vi "zgj地图的构建0911-150原.vi"() -> ()   [LabVIEW 2018]
uses:
  <vilib>/Utility/file.llb/Read Delimited Spreadsheet (string).vi
  <vilib>/vision/NI_Vision_Development_Module.lvlib
panel:
  out "方向":sgl
  out "轨迹跟踪点数":i32
  out "y":dbl
  out "x":dbl
  out "b":dbl[](array[numeric])
  in  "pp":dbl
  out "与目标点的距离":sgl
  in  "guiji":path=path "G:/ICRA-2024-Yuezhen Liu/Labview程序-ICRA2024-YuezhenLiu/small_myRIO_Helmholtz - 1111ke777/zgj轨迹delta为150.txt" caption="call7-8"
  out "i":i32
  out "Image 7":T1(plugin-control)
  in  "Stop (F)":bool
  out "数值 2":dbl
  out "数值":dbl
  out "数组":sgl[](array[numeric])
  out "Objects":T2(array[cluster]) {"Aspect Ratio" format="%.2f"; "Orientation" format="%.2f"; "Area" format="%.2f"; "Object Center"."Y" format="%.2f"; "Object Center"."X" format="%.2f"}
  in  "Settings":T3={"Objects"=0, "Threshold"=128, "Reject Border"=FALSE, "Fill Holes"=FALSE, "Min Object Size"=TRUE, "Min Size"=5000, "Max Object Size"=FALSE, "Max Size"=100, "Show Search Area"=FALSE, "Show Center"=TRUE, "Show Bounding Box"=TRUE} {"Objects" items=["Bright Objects", "Dark Objects"]; "Threshold" min=1 max=999999999 step=1; "Max Size" min=1 max=999999999 step=1; "Min Size" min=1 max=999999999 step=1}
  out "Image 2":T1(plugin-control)
  in  "Range":cluster{"Lower value":sgl, "Upper value":sgl}={"Lower value"=0.0, "Upper value"=128.0} {"Upper value" format="%.2f"; "Lower value" format="%.2f"}
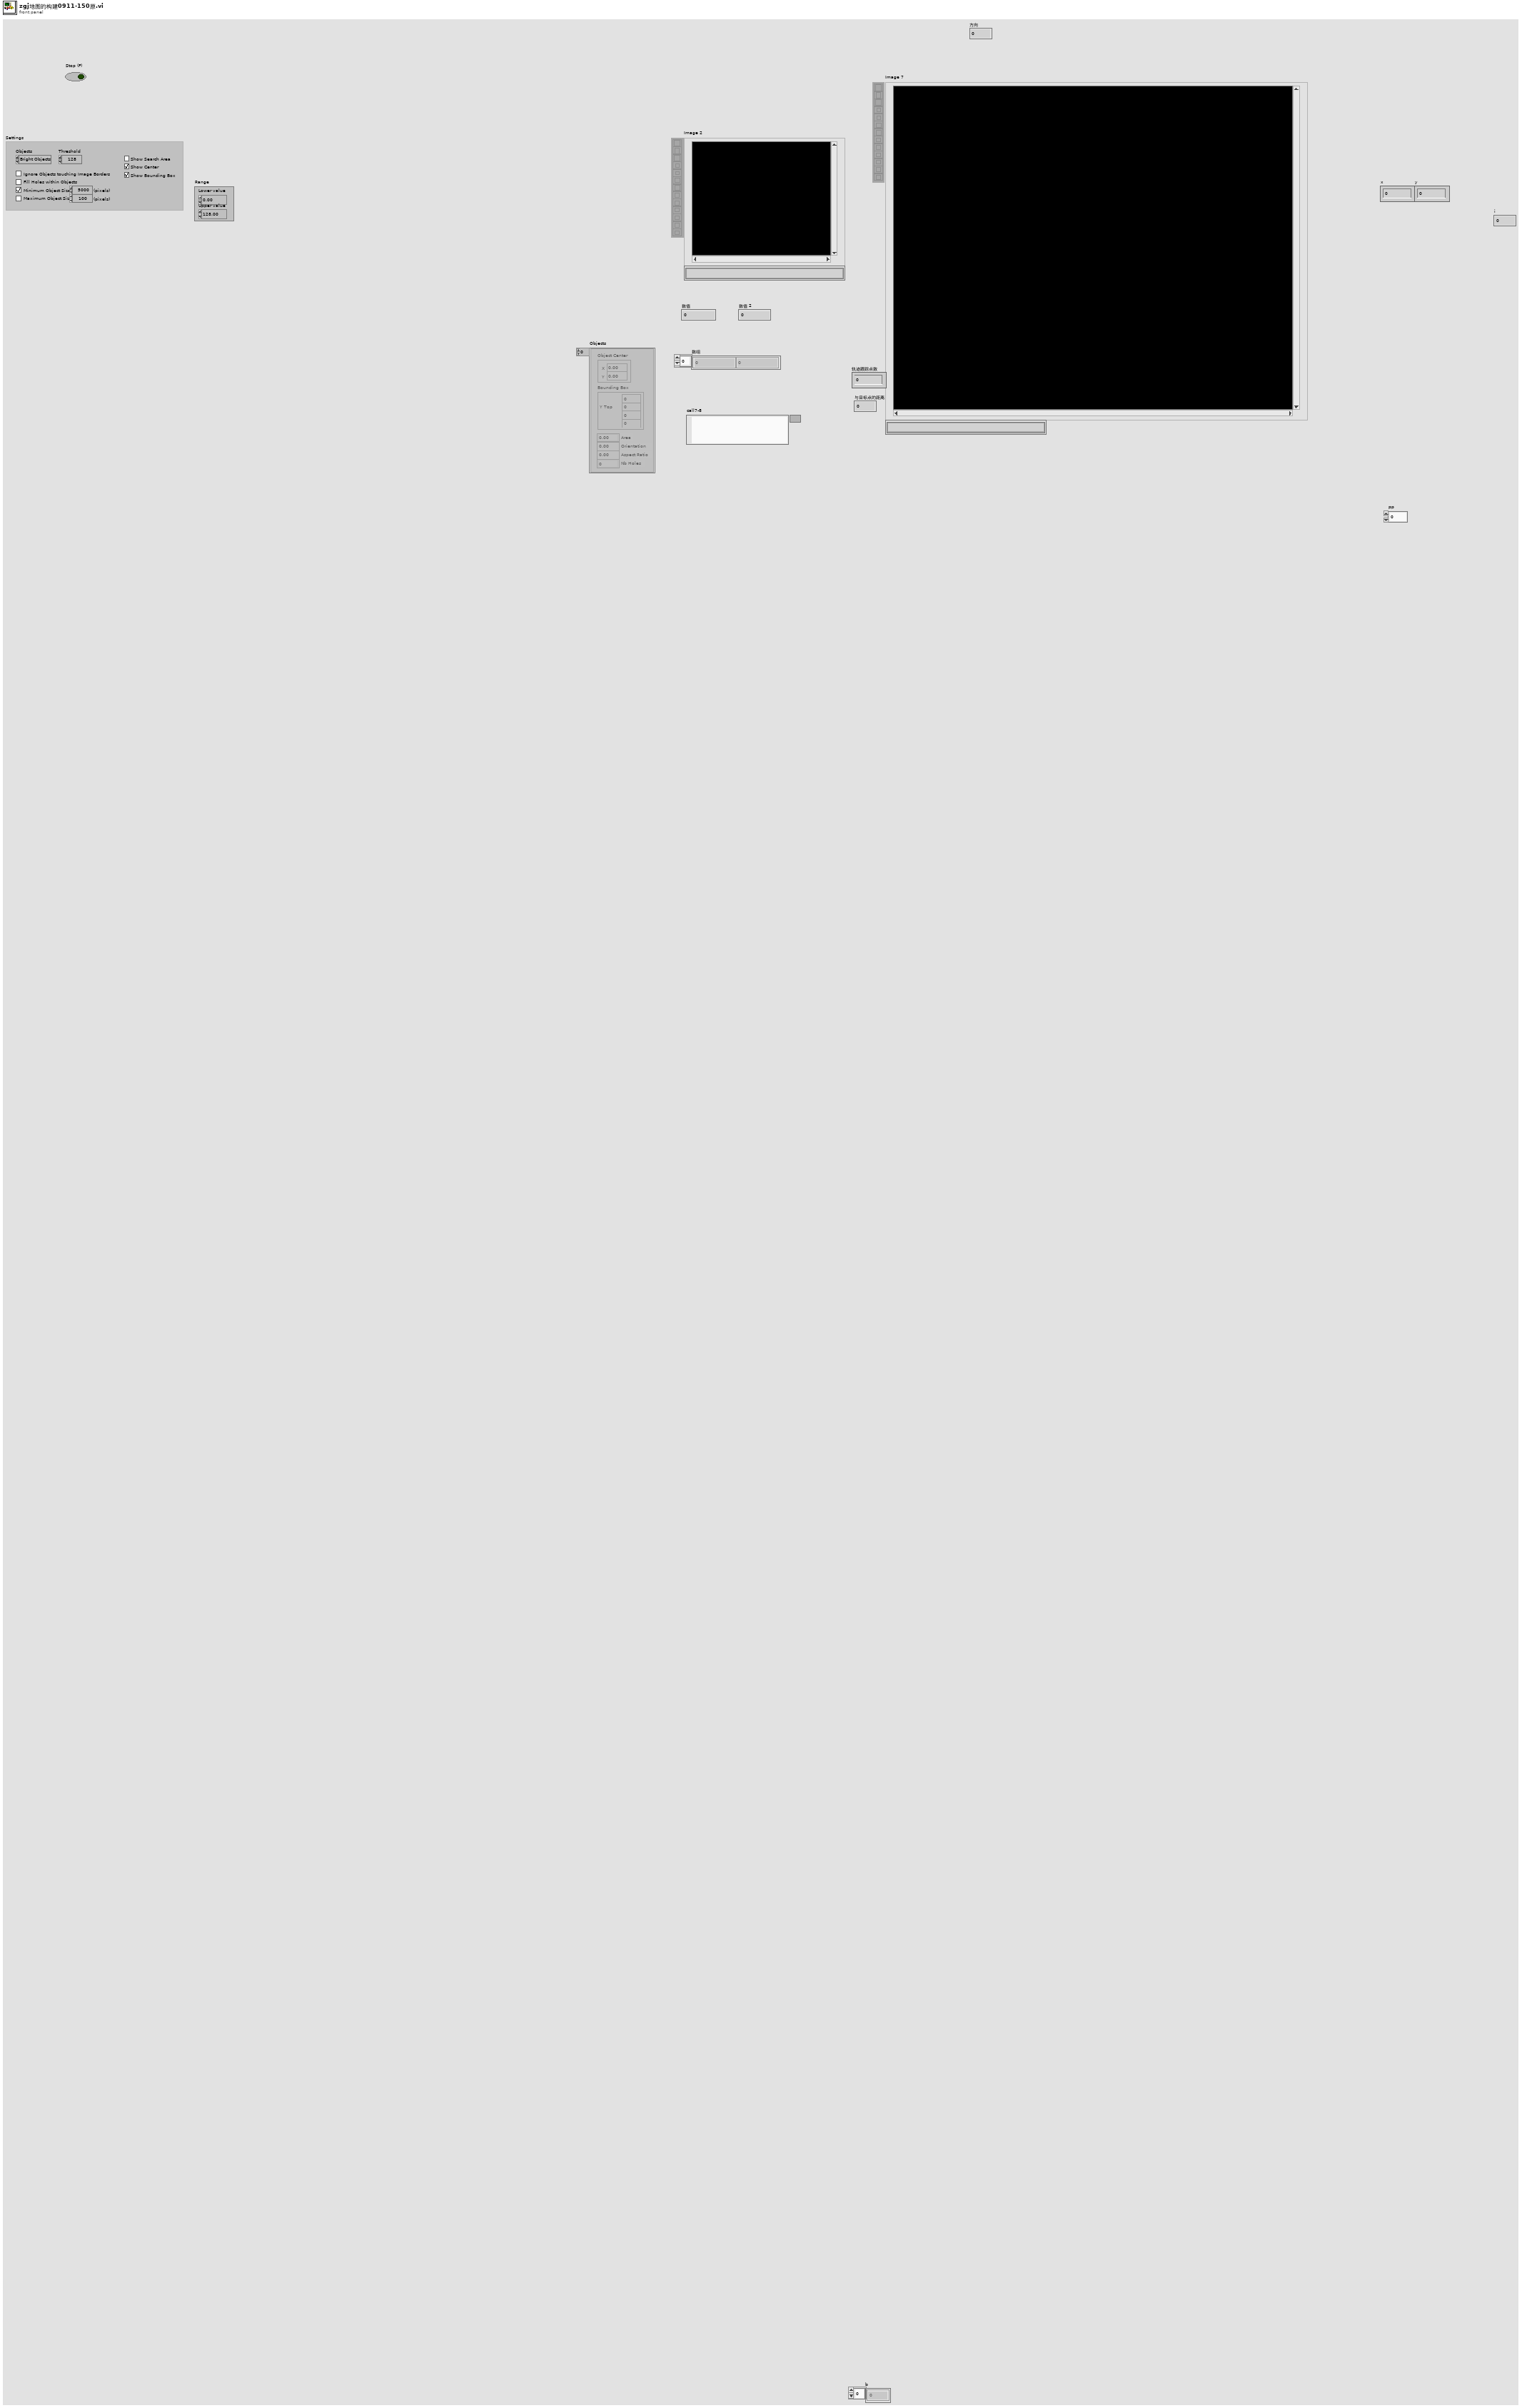
[diagram p1: front panel]
types:
  T1 = typedef "IMAQ Image.ctl" = refnum<image>
  T2 = cluster{"Object Center":cluster{"X":sgl, "Y":sgl}, "Bounding Box":cluster{"X Left":i32, "Y Top":i32, "X Right":i32, "Y Bottom":i32}, "Area":sgl, "Orientation":sgl, "Aspect Ratio":sgl, "Nb Holes":i32}[]
  T3 = cluster{"Objects":u16, "Threshold":i32, "Reject Border":bool, "Fill Holes":bool, "Min Object Size":bool, "Min Size":i32, "Max Object Size":bool, "Max Size":i32, "Show Search Area":bool, "Show Center":bool, "Show Bounding Box":bool}
  T4 = typedef "Image Type" = u32
  T5 = cluster{"Left":i32, "Top":i32, "Right":i32, "Bottom":i32}
  T6 = cluster{"Objects[0]":cluster{"Object Center":cluster{"X":sgl, "Y":sgl}, "Bounding Box":cluster{"X Left":i32, "Y Top":i32, "X Right":i32, "Y Bottom":i32}, "Area":sgl, "Orientation":sgl, "Aspect Ratio":sgl, "Nb Holes":i32}, "Objects[1]":cluster{"Object Center":cluster{"X":sgl, "Y":sgl}, "Bounding Box":cluster{"X Left":i32, "Y Top":i32, "X Right":i32, "Y Bottom":i32}, "Area":sgl, "Orientation":sgl, "Aspect Ratio":sgl, "Nb Holes":i32}, "Objects[2]":cluster{"Object Center":cluster{"X":sgl, "Y":sgl}, "Bounding Box":cluster{"X Left":i32, "Y Top":i32, "X Right":i32, "Y Bottom":i32}, "Area":sgl, "Orientation":sgl, "Aspect Ratio":sgl, "Nb Holes":i32}, "Objects[3]":cluster{"Object Center":cluster{"X":sgl, "Y":sgl}, "Bounding Box":cluster{"X Left":i32, "Y Top":i32, "X Right":i32, "Y Bottom":i32}, "Area":sgl, "Orientation":sgl, "Aspect Ratio":sgl, "Nb Holes":i32}, "Objects[4]":cluster{"Object Center":cluster{"X":sgl, "Y":sgl}, "Bounding Box":cluster{"X Left":i32, "Y Top":i32, "X Right":i32, "Y Bottom":i32}, "Area":sgl, "Orientation":sgl, "Aspect Ratio":sgl, "Nb Holes":i32}, "Objects[5]":cluster{"Object Center":cluster{"X":sgl, "Y":sgl}, "Bounding Box":cluster{"X Left":i32, "Y Top":i32, "X Right":i32, "Y Bottom":i32}, "Area":sgl, "Orientation":sgl, "Aspect Ratio":sgl, "Nb Holes":i32}, "Objects[6]":cluster{"Object Center":cluster{"X":sgl, "Y":sgl}, "Bounding Box":cluster{"X Left":i32, "Y Top":i32, "X Right":i32, "Y Bottom":i32}, "Area":sgl, "Orientation":sgl, "Aspect Ratio":sgl, "Nb Holes":i32}, "Objects[7]":cluster{"Object Center":cluster{"X":sgl, "Y":sgl}, "Bounding Box":cluster{"X Left":i32, "Y Top":i32, "X Right":i32, "Y Bottom":i32}, "Area":sgl, "Orientation":sgl, "Aspect Ratio":sgl, "Nb Holes":i32}, "Objects[8]":cluster{"Object Center":cluster{"X":sgl, "Y":sgl}, "Bounding Box":cluster{"X Left":i32, "Y Top":i32, "X Right":i32, "Y Bottom":i32}, "Area":sgl, "Orientation":sgl, "Aspect Ratio":sgl, "Nb Holes":i32}}
  T7 = cluster{"Object Center":cluster{"X":sgl, "Y":sgl}, "Bounding Box":cluster{"X Left":i32, "Y Top":i32, "X Right":i32, "Y Bottom":i32}, "Area":sgl, "Orientation":sgl, "Aspect Ratio":sgl, "Nb Holes":i32}
  T8 = cluster{"X Left":i32, "Y Top":i32, "X Right":i32, "Y Bottom":i32}
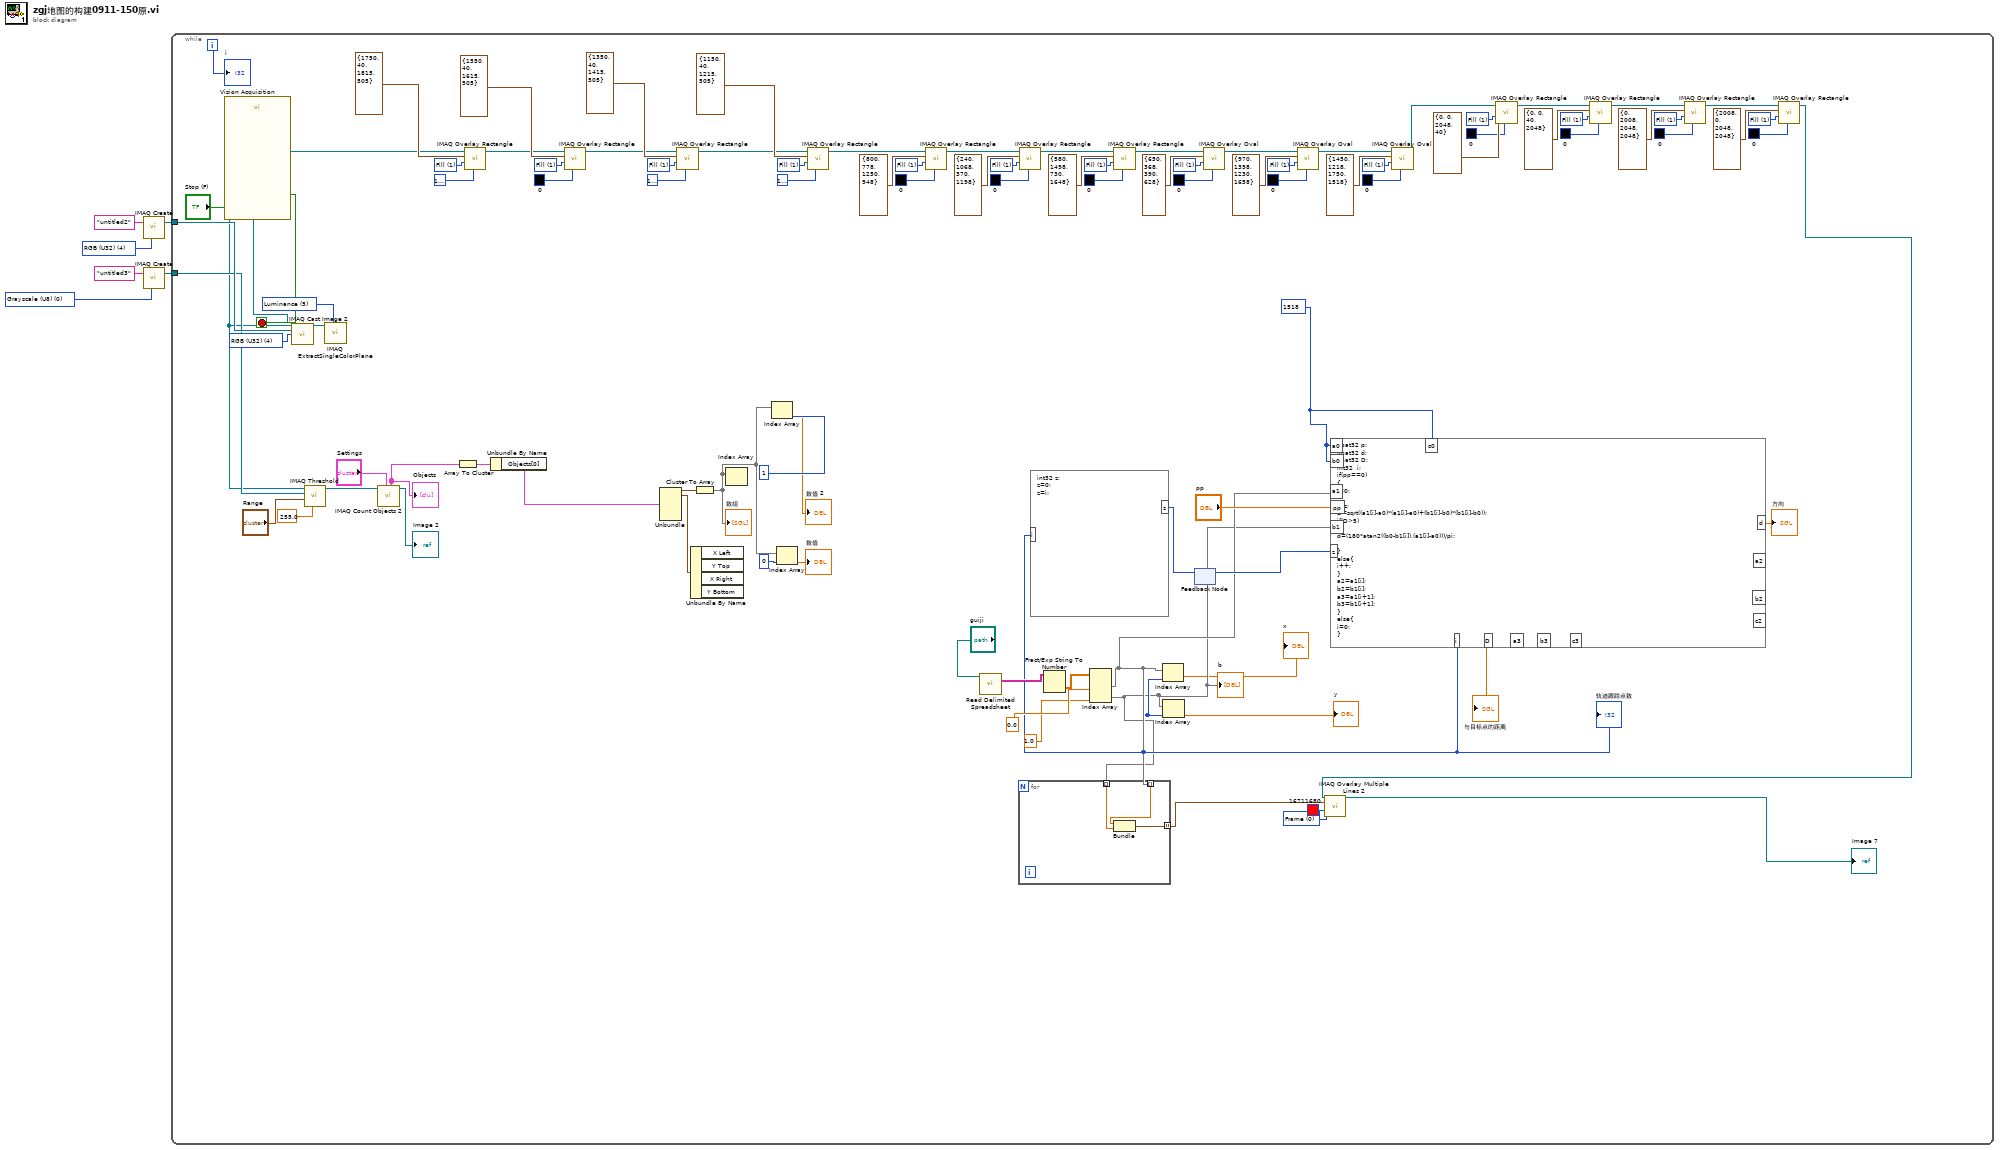
[diagram p0: block diagram]
diagram:
  w1 = T4 0 items=["Grayscale (U8)", "Grayscale (I16)", "Grayscale (SGL)", "Complex (CSG)", "RGB (U32)", "HSL (U32)", "RGB (U64)", "Grayscale (U16)"] ("Image Type")
  w4 = T4 4 items=["Grayscale (U8)", "Grayscale (I16)", "Grayscale (SGL)", "Complex (CSG)", "RGB (U32)", "HSL (U32)", "RGB (U64)", "Grayscale (U16)"] ("Image Type")
  n1 = call "IMAQ Create"("Image Name"="untitled2", "Image Type"=w4) -> ("New Image"=w5:T1)  [unwired: 3 in, 1 out]
  n2 = call "IMAQ Create"("Image Name"="untitled3", "Image Type"=w1) -> ("New Image"=w3:T1)  [unwired: 3 in, 1 out]
  n3 = while {
    tunnel: w5 -> [w107]
    tunnel: w3 -> [w103]
    i -> [w70]
    stop <- w92 stop-if-true
    w8 = u32 0 items=["Frame", "Fill"] ("Drawing Mode (Frame)")
    w13 = 1518 ("Bottom")
    w29 = u32 1 items=["Frame", "Fill", "Highlight"] ("Drawing Mode (Frame)")
    w32 = u32 1 items=["Frame", "Fill", "Highlight"] ("Drawing Mode (Frame)")
    w35 = u32 1 items=["Frame", "Fill", "Highlight"] ("Drawing Mode (Frame)")
    w38 = u32 1 items=["Frame", "Fill", "Highlight"] ("Drawing Mode (Frame)")
    w45 = u32 1 items=["Frame", "Fill"] ("Drawing Mode (Frame)")
    w48 = u32 1 items=["Frame", "Fill"] ("Drawing Mode (Frame)")
    w53 = u32 1 items=["Frame", "Fill"] ("Drawing Mode (Frame)")
    w66 = u32 1 items=["Frame", "Fill", "Highlight"] ("Drawing Mode (Frame)")
    w59 = u32 1 items=["Frame", "Fill"] ("Drawing Mode (Frame)")
    w69 = u32 1 items=["Frame", "Fill", "Highlight"] ("Drawing Mode (Frame)")
    w75 = u32 1 items=["Frame", "Fill", "Highlight"] ("Drawing Mode (Frame)")
    w78 = u32 1 items=["Frame", "Fill", "Highlight"] ("Drawing Mode (Frame)")
    w81 = u32 1 items=["Frame", "Fill", "Highlight"] ("Drawing Mode (Frame)")
    w84 = u32 1 items=["Frame", "Fill", "Highlight"] ("Drawing Mode (Frame)")
    w104 = T4 4 items=["Grayscale (U8)", "Grayscale (I16)", "Grayscale (SGL)", "Complex (CSG)", "RGB (U32)", "HSL (U32)", "RGB (U64)", "Grayscale (U16)"] ("Image Type")
    w106 = 5 items=["Red", "Green", "Blue", "Hue", "Saturation", "Luminance", "Value", "Intensity"] ("Color Plane")
    n4 = call "Vision Acquisition"("Stop (F)"="Stop (F)") -> ("Image Out"=w87:T1, "Stopped"=w92:bool)  [unwired: 24 in, 1 out]
    n5 = call "IMAQ Cast Image 2"("Image Src"=w87, "Image Dst"=w107, "Image Type"=w104) -> ("Image Dst Out"=w105:T1)  [unwired: 11 in, 1 out]
    n6 = call "IMAQ ExtractSingleColorPlane"("Color Plane"=w106, "Image Src"=w105) -> ("Image Dst Out"=w57:T1)  [unwired: 8 in, 1 out]
    n7 = call "IMAQ Threshold"("Replace Value"=sgl 255.0, "Range"="Range", "Image Dst"=w103, "Image Src"=w57) -> ("Image Dst Out"=w85:T1)  [unwired: 6 in, 1 out]
    n8 = call "IMAQ Count Objects 2"("Settings"="Settings", "Image"=w85) -> ("Image Out"=→"Image 2":T1, "Objects"=w99:T2)  [unwired: 5 in, 3 out]
    "Objects" <- w99
    n9 = Array To Cluster(array=w99) -> (cluster=w98:T6)
    n10 = call "IMAQ Overlay Rectangle"("Color"=u32 16777222, "Drawing Mode (Frame)"=w78, "Rectangle"=T5 {"Left"=1750, "Top"=40, "Right"=1815, "Bottom"=505}, "Image"=w57) -> ("Image Out"=w56:T1)  [unwired: 6 in, 1 out]
    n11 = Unbundle By Name(w98) -> ("Objects[0]"=w97:T7)
    n12 = call "IMAQ Overlay Rectangle"("Color"=u32 0, "Drawing Mode (Frame)"=w75, "Rectangle"=T5 {"Left"=1550, "Top"=40, "Right"=1615, "Bottom"=505}, "Image"=w56) -> ("Image Out"=w72:T1)  [unwired: 6 in, 1 out]
    n13 = Unbundle(w97) -> ("Object Center"=w96:cluster{"X":sgl, "Y":sgl}, "Bounding Box"=w86:T8)  [unwired: 4 out]
    n14 = call "IMAQ Overlay Rectangle"("Color"=u32 16777222, "Drawing Mode (Frame)"=w81, "Rectangle"=T5 {"Left"=1350, "Top"=40, "Right"=1415, "Bottom"=505}, "Image"=w72) -> ("Image Out"=w71:T1)  [unwired: 6 in, 1 out]
    n15 = Unbundle By Name(w86) -> ()  [unwired: 4 out]
    n16 = Cluster To Array(cluster=w96) -> (array=w94:sgl[])
    "数组" <- w94
    n17 = Index Array(array=w94) -> ()  [unwired: 1 in, 1 out]
    n18 = Index Array(array=w94, index=1 ("索引")) -> (element=→"数值 2":sgl)
    n19 = Index Array(array=w94, index=0 ("索引")) -> (element=→"数值":sgl)
    n20 = call "IMAQ Overlay Rectangle"("Color"=u32 16777222, "Drawing Mode (Frame)"=w84, "Rectangle"=T5 {"Left"=1150, "Top"=40, "Right"=1215, "Bottom"=505}, "Image"=w71) -> ("Image Out"=w58:T1)  [unwired: 6 in, 1 out]
    n21 = call "IMAQ Overlay Rectangle"("Color"=u32 0, "Drawing Mode (Frame)"=w69, "Rectangle"=T5 {"Left"=800, "Top"=778, "Right"=1250, "Bottom"=948}, "Image"=w58) -> ("Image Out"=w62:T1)  [unwired: 6 in, 1 out]
    n22 = call-poly <vilib>:"Read Delimited Spreadsheet.vi"("file path (dialog if empty)"="guiji") -> ("all rows"=w26:string[][])  [unwired: 9 in, 5 out]
    n23 = call "IMAQ Overlay Rectangle"("Color"=u32 0, "Drawing Mode (Frame)"=w59, "Rectangle"=T5 {"Left"=240, "Top"=1068, "Right"=370, "Bottom"=1198}, "Image"=w62) -> ("Image Out"=w63:T1)  [unwired: 6 in, 1 out]
    n24 = Fract/Exp String To Number(string=w26) -> (number=w25:dbl[][])  [unwired: 3 in, 1 out]
    n25 = Index Array(array=w25, index (col) #1=0.0, index (col) #2=1.0) -> (element #1=w18:dbl[], element #2=w16:dbl[])  [unwired: 2 in]
    "b" <- w16
    n26 = for {
      tunnel: w18 -> [w110] mode=indexing
      tunnel: w16 -> [w109] mode=indexing
      tunnel: [w108] -> w12 mode=indexing
      n27 = Bundle("String"=w110, "String"=w109) -> (w108:cluster{"String":dbl, "String":dbl})  [unwired: 1 in]
    }
    n28 = call "IMAQ Overlay Rectangle"("Color"=u32 0, "Drawing Mode (Frame)"=w66, "Rectangle"=T5 {"Left"=580, "Top"=1498, "Right"=730, "Bottom"=1648}, "Image"=w63) -> ("Image Out"=w55:T1)  [unwired: 6 in, 1 out]
    n29 = feedback #1() -> (w21:i32)  [unwired: 1 in]
    n30 = call "IMAQ Overlay Oval"("Color"=u32 0, "Drawing Mode (Frame)"=w53, "Bounding Rectangle"=T5 {"Left"=650, "Top"=368, "Right"=390, "Bottom"=628}, "Image"=w55) -> ("Image Out"=w50:T1)  [unwired: 6 in, 1 out]
    n31 = call "IMAQ Overlay Oval"("Color"=u32 0, "Drawing Mode (Frame)"=w48, "Bounding Rectangle"=T5 {"Left"=970, "Top"=1398, "Right"=1230, "Bottom"=1658}, "Image"=w50) -> ("Image Out"=w51:T1)  [unwired: 6 in, 1 out]
    n32 = formula code="float32 p;\nfloat32 d;\nfloat32 D;\nint32  i;\nif(pp==0)\n{\ni=0;\n\ni=z;\nD=sqrt((a1[i]-a0)*(a1[i]-a0)+(b1[i]-b0)*(b1[i]-b0));\nif(D>5)\n{\nd=(180*atan2((b0-b1[i]),(a1[i]-a0)))/pi;\n\n}\nelse{\ni++;\n}\na2=a1[i];\nb2=b1[i];\na3=a1[i+1];\nb3=b1[i+1];\n}\nelse{\ni=0;\n}"("a0"=w13, "b0"=w13, "a1"=w18, "b1"=w16, "z"=w21, "pp"="pp", "c0"=w13) -> ("i"=w17:i32, "D"=→"与目标点的距离":sgl, "d"=→"方向":sgl)  [unwired: 6 out]
    "轨迹跟踪点数" <- w17
    n33 = formula code="int32 z;\nz=0;\nz=i;"("i"=w17) -> ("z"=w22:i32)
    n34 = Index Array(array=w18, index=w17) -> (element=→"x":dbl)
    n35 = Index Array(array=w16, index=w17) -> (element=→"y":dbl)
    n36 = feedback-in #1(w22) -> ()
    n37 = call "IMAQ Overlay Oval"("Color"=u32 0, "Drawing Mode (Frame)"=w45, "Bounding Rectangle"=T5 {"Left"=1450, "Top"=1218, "Right"=1750, "Bottom"=1518}, "Image"=w51) -> ("Image Out"=w43:T1)  [unwired: 6 in, 1 out]
    n38 = call "IMAQ Overlay Rectangle"("Color"=u32 0, "Drawing Mode (Frame)"=w38, "Rectangle"=T5 {"Left"=0, "Top"=0, "Right"=2048, "Bottom"=40}, "Image"=w43) -> ("Image Out"=w42:T1)  [unwired: 6 in, 1 out]
    n39 = call "IMAQ Overlay Rectangle"("Color"=u32 0, "Drawing Mode (Frame)"=w35, "Rectangle"=T5 {"Left"=0, "Top"=0, "Right"=40, "Bottom"=2048}, "Image"=w42) -> ("Image Out"=w41:T1)  [unwired: 6 in, 1 out]
    n40 = call "IMAQ Overlay Rectangle"("Color"=u32 0, "Drawing Mode (Frame)"=w32, "Rectangle"=T5 {"Left"=0, "Top"=2008, "Right"=2048, "Bottom"=2048}, "Image"=w41) -> ("Image Out"=w40:T1)  [unwired: 6 in, 1 out]
    n41 = call "IMAQ Overlay Rectangle"("Color"=u32 0, "Drawing Mode (Frame)"=w29, "Rectangle"=T5 {"Left"=2008, "Top"=0, "Right"=2048, "Bottom"=2048}, "Image"=w40) -> ("Image Out"=w11:T1)  [unwired: 6 in, 1 out]
    n42 = call "IMAQ Overlay Multiple Lines 2"("Image"=w11, "Line End Points"=w12, "Drawing Mode (Frame)"=w8, "Color"=u32 16711680) -> ("Image Out"=→"Image 7":T1)  [unwired: 10 in, 1 out]
    "i" <- w70
  }
